vi "Quick Display Wave.vi"(8 "waveform":i32, 11 "EODDataIn":T1(array[cluster])) -> (3 "Waveform Chart":waveform(dbl)(graph))   [LabVIEW 2014]
panel:
  # "Quick Display Wave VI"
  # "Inputs"
  # "Outputs"
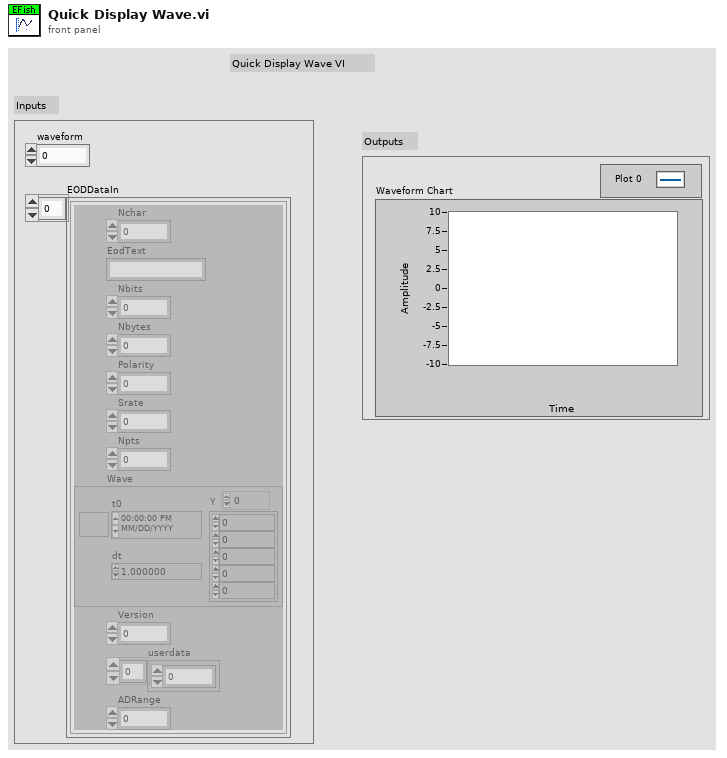
[diagram p1: front panel]
types:
  T1 = cluster{"Nchar":i32, "EodText":string, "Nbits":i32, "Nbytes":i32, "Polarity":i32, "Srate":i32, "Npts":i32, "Wave":waveform(dbl), "Version":i32, "userdata":dbl[], "ADRange":dbl}[]
  T2 = cluster{"Nchar":i32, "EodText":string, "Nbits":i32, "Nbytes":i32, "Polarity":i32, "Srate":i32, "Npts":i32, "Wave":waveform(dbl), "Version":i32, "userdata":dbl[], "ADRange":dbl}
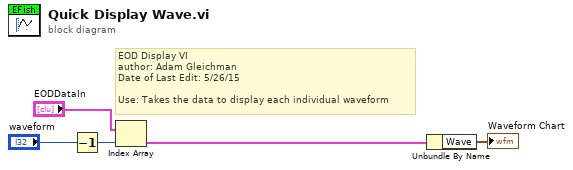
[diagram p0: block diagram]
diagram:
  # "EOD Display VI\nauthor: Adam Gleichman\nDate of Last Edit: 5/26/15\n\nUse: Takes the data to display each individual waveform"
  n1 = Decrement(x="waveform") -> (x-1=w1:i32)
  n2 = Index Array(array="EODDataIn", index=w1) -> (element=w4:T2)
  n3 = Unbundle By Name(w4) -> ("Wave"=→"Waveform Chart":waveform(dbl))
